vi "SLL DE Remove Empty Elements (Device) from array.vi"(9 "Channel ArrayIn":cluster{"Device Channel List":string[]}[](array[cluster]), 10 "Devices Names In":string[](array[string])) -> (1 "Channel Array Out":cluster{"Device Channel List":string[]}[](array[cluster]), 2 "Devices Names":string[](array[string]))   [LabVIEW 2013]
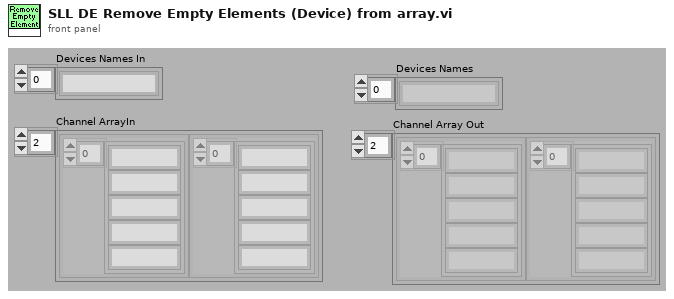
[diagram p1: front panel]
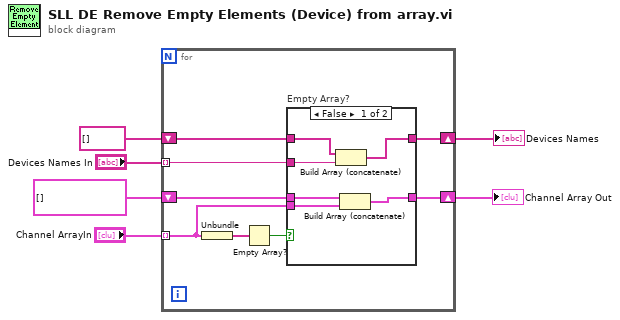
[diagram p0: block diagram]
diagram:
  n1 = for {
    tunnel: "Channel ArrayIn" -> [w12] mode=indexing
    shift-right: [w11] -> w5
    shift-left: cluster{"Device Channel List":string[]}[] [] -> [w10]
    tunnel: "Devices Names In" -> [w9] mode=indexing
    shift-right: [w7] -> w1
    shift-left: string[] [] ("Device Channel List") -> [w8]
    n2 = Unbundle(w12) -> ("Device Channel List"=w14:string[])
    n3 = Empty Array?(array=w14) -> (empty?=w13:bool)
    n4 = case "Empty Array?" shown="False" w13 {
      tunnel: w12 -> [w20 _]
      tunnel: [w19 w22] -> w11
      tunnel: w10 -> [w18 w22]
      tunnel: w9 -> [w17 _]
      tunnel: w8 -> [w16 w21]
      tunnel: [w15 w21] -> w7
      frame False {
        n5 = Build Array (concatenate)(w16, w17) -> (w15:string[])
        n6 = Build Array (concatenate)(w18, w20) -> (w19:cluster{"Device Channel List":string[]}[])
      }
      frame True {
      }
    }
  }
  "Channel Array Out" <- w5
  "Devices Names" <- w1
